vi "Encode repeated string.vi"(7 "Field Number":i32, 10 "string":string[](array[string]), 11 "Buffer in":u8[](array[numeric]) format="%.0x") -> (3 "Buffer":u8[](array[numeric]) format="%.0x")   [LabVIEW 2020, in "LV-Proto.lvlib"]
uses:
  LV-Proto.lvlib
  Encode bytes.vi
  Wire Encode Tag.vi
  Encode LEN.vi
  Wire Encode Varint I32.vi
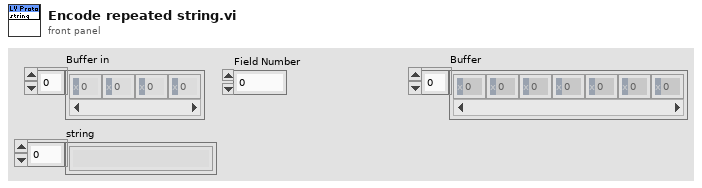
[diagram p1: front panel]
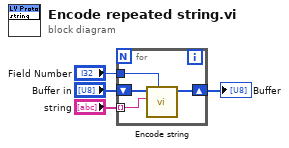
[diagram p0: block diagram]
diagram:
  n1 = for {
    shift-right: [w5] -> w1
    shift-left: "Buffer in" -> [w8]
    tunnel: "string" -> [w6] mode=indexing
    tunnel: "Field Number" -> [w7]
    n2 = call "Encode string.vi"("Field Number"=w7, "string"=w6, "Buffer in"=w8) -> ("Buffer"=w5:u8[])  [unwired: 8 in]
  }
  "Buffer" <- w1
